vi "Ammeter Measure.vi"(8 "error in (no error)":errorcluster, 11 "VISA resource name in":refnum<visa-resource-name>) -> (0 "error out":errorcluster, 2 "Measurement":dbl, 3 "VISA resource name out":refnum<visa-resource-name>)   [LabVIEW 2016, in "Hall Effect Library.lvlib"]
uses:
  Hall Effect Library.lvlib
  Global Variables/Instruments.vi
  Ammeter Measure (None).vi
  Ammeter Measure (648X).vi
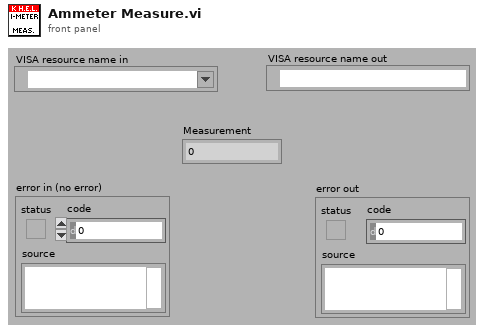
[diagram p1: front panel]
types:
  T1 = typedef "Hall Effect Library.lvlib/Ammeters.ctl" = enum16{"None", "648X"}
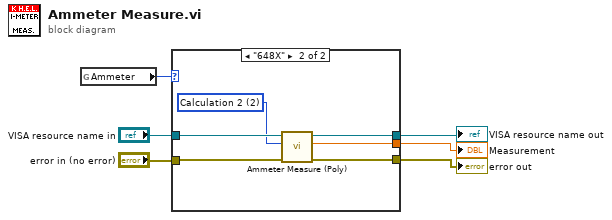
[diagram p0: block diagram]
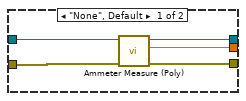
[diagram p2: hidden frame]
diagram:
  n1 = global read "Instruments.vi" "Ammeter"() -> (w6:T1)
  n2 = case shown="\"648X\"" w6 {
    tunnel: "VISA resource name in" -> [w11 w16]
    tunnel: [w10 w15] -> w4
    tunnel: "error in (no error)" -> [w9 w13]
    tunnel: [w8 w17] -> w2
    tunnel: [w7 w14] -> w3
    frame "None", Default {
      n3 = call-poly "Ammeter Measure (Poly).vi"("error in (no error)"=w9, "VISA resource name in"=w11) -> ("error out"=w8:errorcluster, "Measurement"=w7:dbl, "VISA resource name out"=w10:refnum<visa-resource-name>)  [unwired: 7 out]
    }
    frame "648X" {
      w12 = u16 2 items=["Function", "Calculation 1", "Calculation 2", "Calculation 3"] ("Source (Function)")
      n4 = call-poly "Ammeter Measure (Poly).vi"("error in (no error)"=w13, "Source (Function)"=w12, "VISA resource name in"=w16) -> ("error out"=w17:errorcluster, "Measurement"=w14:dbl, "VISA resource name out"=w15:refnum<visa-resource-name>)  [unwired: 6 out]
    }
  }
  "error out" <- w2
  "VISA resource name out" <- w4
  "Measurement" <- w3
